vi "python script test.vi"() -> ()   [LabVIEW 2014]
panel:
  out "standard output 2":string
  out "standard error 2":string
  out "error out 2":errorcluster
  in  "get-temperature":bool
  in  "send":bool
  in  "stop":bool
  in  "display text":string=" Wizzo"
  out "error out":errorcluster
  out "standard error":string
  out "standard output":string
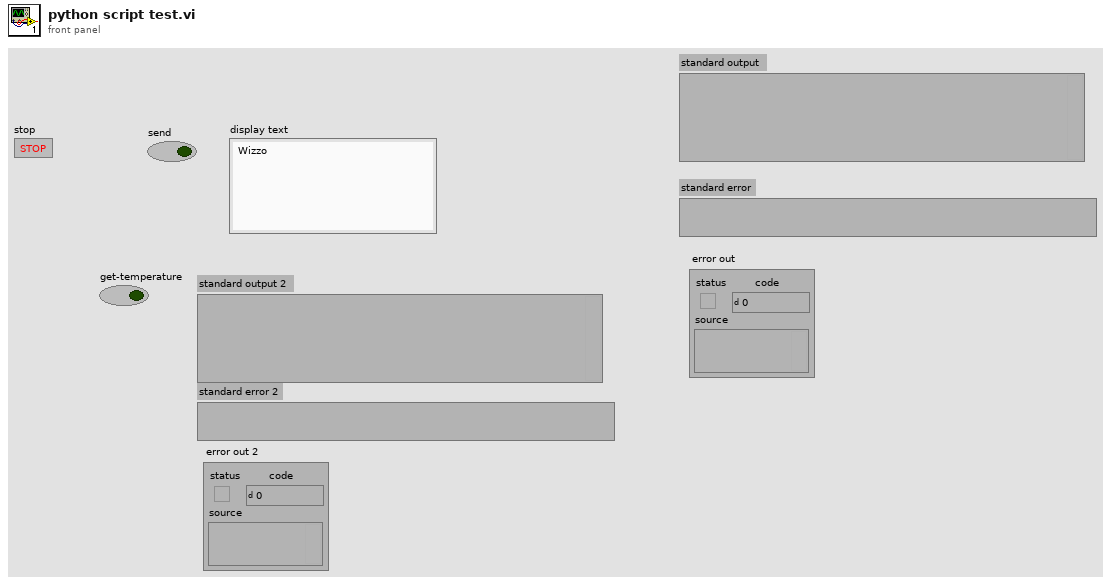
[diagram p1: front panel]
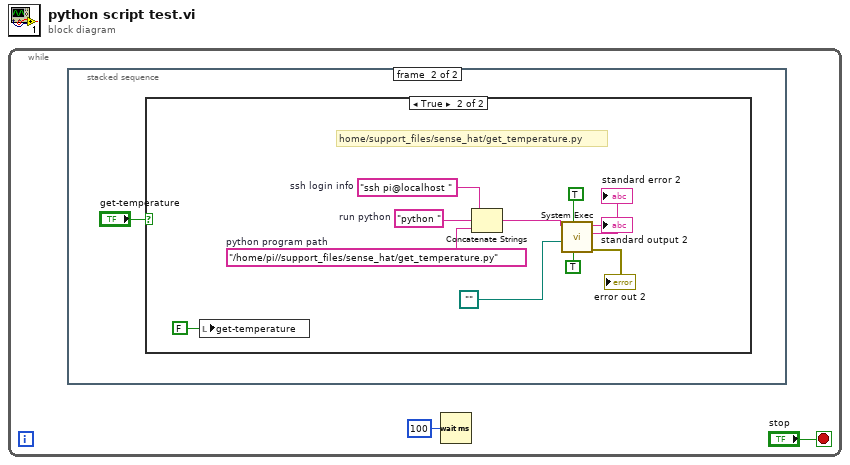
[diagram p0: block diagram]
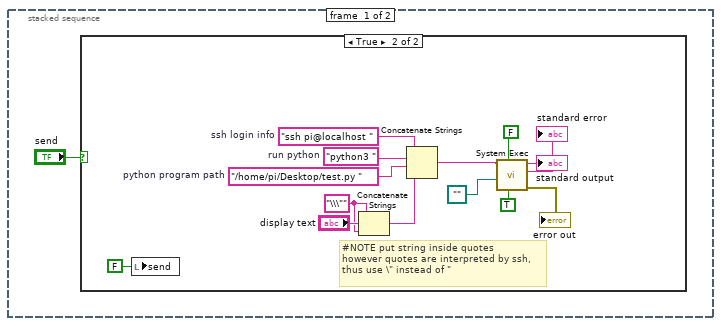
[diagram p2: hidden frame]
diagram:
  n1 = while {
    stop <- "stop" stop-if-true
    n2 = stacked-sequence {
      frame #0 {
        n3 = case shown="True" "send" {
          frame False {
          }
          frame True {
            w4 = "\\\"" ("string")
            w9 = "ssh pi@localhost "  # ssh login info
            w8 = "/home/pi/Desktop/test.py "  # python program path
            w15 = "python3 "  # run python
            # "#NOTE put string inside quotes\nhowever quotes are interpreted by ssh,\nthus use \\\" instead of \""
            n4 = local write "send"(FALSE ("send")) -> ()
            n5 = Concatenate Strings(w4, "display text", w4) -> (w5:string)
            n6 = Concatenate Strings(w9, w15, w8, w5) -> (w10:string)
            n7 = call <vilib>:"System Exec.vi"("run minimized? (F)"=TRUE, "wait until completion? (T)"=FALSE, "working directory"=path "", "command line"=w10) -> ("error out"=→"error out":errorcluster, "standard error"=→"standard error":string, "standard output"=→"standard output":string)  [unwired: 4 in, 1 out]
          }
        }
      }
      frame #1 {
        n8 = case shown="True" "get-temperature" {
          frame False {
          }
          frame True {
            w19 = "ssh pi@localhost "  # ssh login info
            w20 = "/home/pi//support_files/sense_hat/get_temperature.py"  # python program path
            w21 = "python "  # run python
            # "home/support_files/sense_hat/get_temperature.py"
            n9 = local write "get-temperature"(FALSE ("send")) -> ()
            n10 = Concatenate Strings(w19, w21, w20) -> (w23:string)
            n11 = call <vilib>:"System Exec.vi"("run minimized? (F)"=TRUE, "wait until completion? (T)"=TRUE, "working directory"=path "", "command line"=w23) -> ("error out"=→"error out 2":errorcluster, "standard error"=→"standard error 2":string, "standard output"=→"standard output 2":string)  [unwired: 4 in, 1 out]
          }
        }
      }
    }
    n12 = Wait (ms)(milliseconds to wait=u32 100) -> ()  [unwired: 1 out]
  }
